vi "test - Read Paired Tunnels.vi"(8 "error in (no error)":errorcluster, 11 "TestCase in":refnum<class "testcase-csmhelper.lvclass">) -> (0 "error out":errorcluster, 3 "TestCase out":refnum<class "testcase-csmhelper.lvclass">)   [LabVIEW 2017, in "testcase-csmhelper.lvclass"]
uses:
  testcase-csmhelper.lvclass
  src/user.lib/_NEVSTOP/Communicable State Machine(CSM)/_csmHelper/CSM-Helper.lvclass/CSM-Helper.ctl
  src/user.lib/_NEVSTOP/Communicable State Machine(CSM)/_csmHelper/Properties/Read VI Ref.vi
  src/user.lib/_NEVSTOP/Communicable State Machine(CSM)/_csmHelper/API/Create From VI Reference.vi
  src/user.lib/_NEVSTOP/Communicable State Machine(CSM)/_csmHelper/API/Start Undo.vi
  src/user.lib/_NEVSTOP/Communicable State Machine(CSM)/_csmHelper/API/Add State Frame.vi
  src/user.lib/_NEVSTOP/Communicable State Machine(CSM)/_csmHelper/API/Connect Paired Tunnels.vi
  src/user.lib/_NEVSTOP/Communicable State Machine(CSM)/_csmHelper/API/Stop Undo.vi
  src/user.lib/_NEVSTOP/Communicable State Machine(CSM)/_csmHelper/API/Undo.vi
  src/user.lib/_NEVSTOP/Communicable State Machine(CSM)/_csmHelper/API/Destroy.vi
  <vilib>/addons/_JKI Toolkits/VI Tester/TestCase.llb/TestCase.lvclass
  src/user.lib/_NEVSTOP/Communicable State Machine(CSM)/_csmHelper/CSM-Helper.lvclass
  C:/Program Files (x86)/National Instruments/LabVIEW 2017/vi.lib/addons/_JKI Toolkits/VI Tester/TestCase.llb/TestCase.lvclass
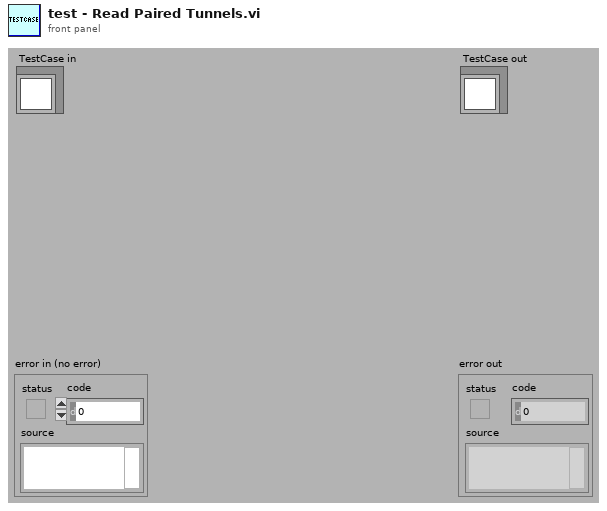
[diagram p1: front panel]
types:
  T1 = enum32{"Bad", "Idle", "Run top level", "Running"}
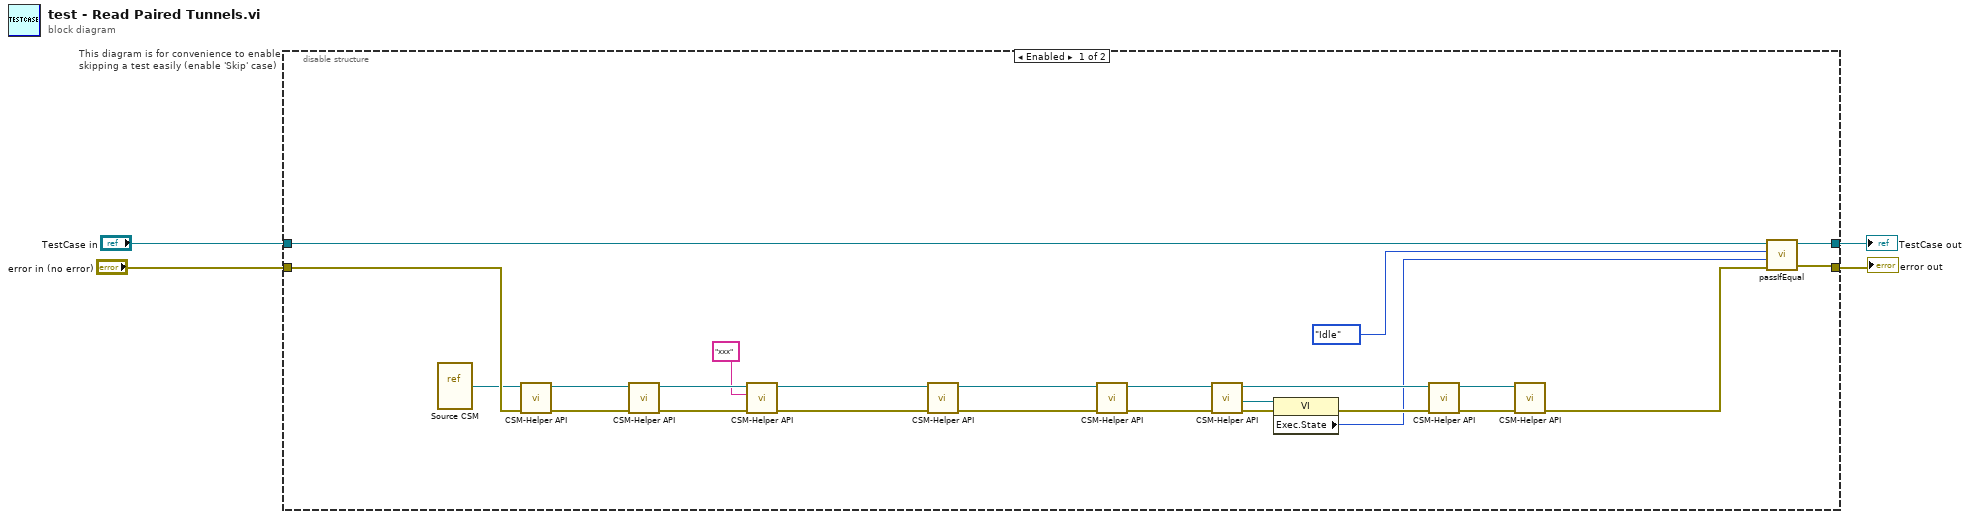
[diagram p0: block diagram]
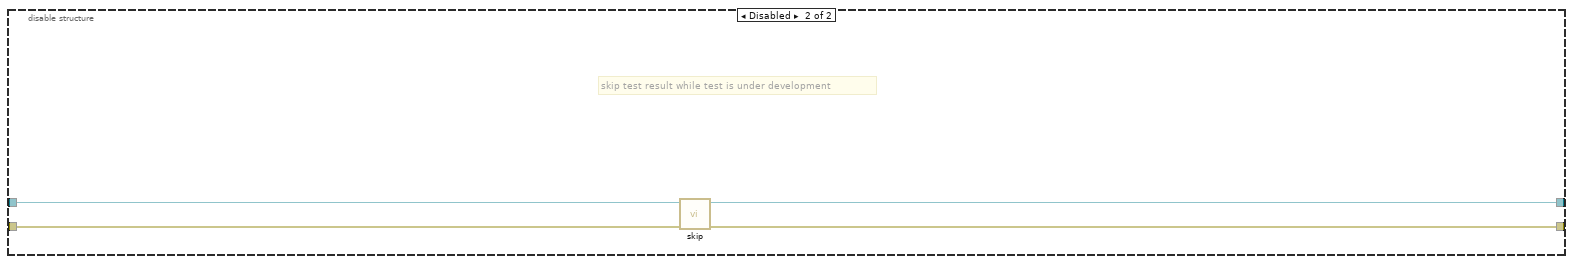
[diagram p2: hidden frame]
diagram:
  n1 = disable-structure "This diagram is for convenience to enable skipping a test easily (enable 'Skip' case)" shown="Enabled" {
    disable-tunnel: "TestCase in" -> [w29 w33]
    disable-tunnel: [w28 w31] -> w1
    disable-tunnel: [w27 w32] -> w3
    disable-tunnel: "error in (no error)" -> [w9 w30]
    frame Enabled {
      n2 = vi-ref "Source CSM.vi"() -> (w5:refnum<vi>)
      n3 = call-poly "CSM-Helper API.vi"("error in (no error)"=w9, "VI"=w5) -> ("error out"=w23:errorcluster, "CSM-Helper.lvclass"=w22:refnum<class "CSM-Helper.lvclass">)  [unwired: 8 in]
      n4 = call-poly "CSM-Helper API.vi"("error in (no error)"=w23, "CSM-Helper in"=w22) -> ("error out"=w21:errorcluster, "CSM-Helper out"=w19:refnum<class "CSM-Helper.lvclass">)  [unwired: 8 in]
      n5 = call-poly "CSM-Helper API.vi"("error in (no error)"=w21, "element"="xxx", "CSM-Helper in"=w19) -> ("error out"=w20:errorcluster, "CSM-Helper out"=w18:refnum<class "CSM-Helper.lvclass">)  [unwired: 6 in, 1 out]
      n6 = call-poly "CSM-Helper API.vi"("error in (no error)"=w20, "CSM-Helper in"=w18) -> ("error out"=w26:errorcluster, "CSM-Helper out"=w25:refnum<class "CSM-Helper.lvclass">)  [unwired: 8 in]
      n7 = call-poly "CSM-Helper API.vi"("error in (no error)"=w26, "CSM-Helper in"=w25) -> ("error out"=w24:errorcluster, "CSM-Helper out"=w15:refnum<class "CSM-Helper.lvclass">)  [unwired: 8 in]
      n8 = call-poly "CSM-Helper API.vi"("error in (no error)"=w24, "CSM-Helper in"=w15) -> ("error out"=w16:errorcluster, "VI"=w13:refnum<vi>, "CSM-Helper out"=w10:refnum<class "CSM-Helper.lvclass">)  [unwired: 7 in]
      n9 = property class="VI"(reference=w13, error in=w16) -> (error out=w14:errorcluster, "Exec.State"=w7:T1)  [unwired: 1 out]
      n10 = call-poly "CSM-Helper API.vi"("error in (no error)"=w14, "CSM-Helper in"=w10) -> ("error out"=w12:errorcluster, "CSM-Helper out"=w11:refnum<class "CSM-Helper.lvclass">)  [unwired: 8 in]
      n11 = call-poly "CSM-Helper API.vi"("error in (no error)"=w12, "CSM-Helper in"=w11) -> ("error out"=w8:errorcluster)  [unwired: 8 in, 1 out]
      n12 = call-dynamic "passIfEqual.vi"("error in (no error)"=w8, "y"=w7, "x"=T1."Idle", "TestCase in"=w29) -> ("error out"=w27:errorcluster, "TestCase out"=w28:refnum<class "testcase-csmhelper.lvclass">)  [unwired: 6 in]
    }
    frame Disabled {
      # "skip test result while test is under development"
      n13 = call <vilib>:"skip.vi"("error in (no error)"=w30, "TestCase in"=w33) -> ("error out"=w32:errorcluster, "TestCase out"=w31:refnum<class "testcase-csmhelper.lvclass">)  [unwired: 8 in]
    }
  }
  "error out" <- w3
  "TestCase out" <- w1
